vi "main.vi"() -> ()   [LabVIEW 2010]
uses:
  <vilib>/Platform/TimedLoop/XDataNode/XDataNode.xnode
  <vilib>/Platform/TimedLoop/XDataNode/nitl_modes.ctl
  <vilib>/Platform/TimedLoop/XDataNode/XDNodeRunTimeDep.lvlib
  <vilib>/Platform/TimedLoop/XDataNode/wakeup.ctl
  <vilib>/Platform/TimedLoop/XDataNode/timing_clust.ctl
  <vilib>/eio/EIONode/EIONode.xnode
  common_typedefs/DAC_channel_enable_cluster.ctl
  common_typedefs/DAC_voltage_cluster.ctl
  common_typedefs/DAC_values_cluster.ctl
panel:
  in  "converter box version":i16=2 min=1 max=2
  out "current DAQ values":T1={"DAC channel enable"={"ch0"=TRUE, "ch1"=TRUE, "ch2"=TRUE, "ch3"=TRUE, "ch4"=TRUE, "ch5"=TRUE, "ch6"=TRUE}, "DAC voltage"={"ch0"=0, "ch1"=0, "ch2"=0, "ch3"=0, "ch4"=0, "ch5"=0, "ch6"=0}, "offset"=0, "channel index"=0, "bit index"=0, "synch?"=FALSE, "DAC clock"=FALSE, "finished?"=FALSE} {"bit index" min=-1 max=17 step=1; "channel index" max=7 step=1; "offset" max=4095; "DAC voltage"."ch6" max=4095 step=1; "DAC voltage"."ch5" max=4095 step=1; "DAC voltage"."ch4" max=4095 step=1; "DAC voltage"."ch3" max=4095 step=1; "DAC voltage"."ch2" max=4095 step=1; "DAC voltage"."ch1" max=4095 step=1; "DAC voltage"."ch0" max=4095 step=1}
  in  "DAC values in":T1={"DAC channel enable"={"ch0"=TRUE, "ch1"=TRUE, "ch2"=TRUE, "ch3"=TRUE, "ch4"=TRUE, "ch5"=TRUE, "ch6"=TRUE}, "DAC voltage"={"ch0"=0, "ch1"=0, "ch2"=0, "ch3"=0, "ch4"=0, "ch5"=0, "ch6"=0}, "offset"=0, "channel index"=0, "bit index"=0, "synch?"=FALSE, "DAC clock"=FALSE, "finished?"=FALSE} {"bit index" min=-1 max=17 step=1; "channel index" max=7 step=1; "offset" max=4095; "DAC voltage"."ch6" max=4095 step=1; "DAC voltage"."ch5" max=4095 step=1; "DAC voltage"."ch4" max=4095 step=1; "DAC voltage"."ch3" max=4095 step=1; "DAC voltage"."ch2" max=4095 step=1; "DAC voltage"."ch1" max=4095 step=1; "DAC voltage"."ch0" max=4095 step=1}
  in  "dataAndControlResetButton":bool
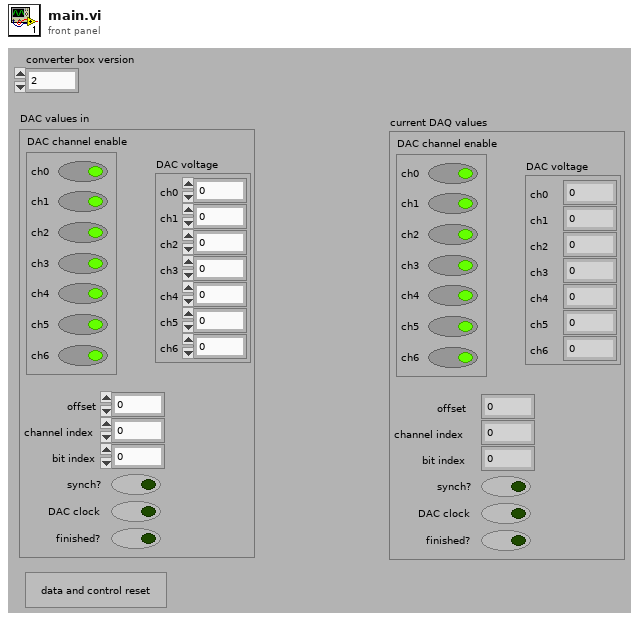
[diagram p1: front panel]
types:
  T1 = typedef "DAC_values_cluster.ctl" = cluster{"DAC channel enable":T2, "DAC voltage":T3, "offset":u16, "channel index":u16, "bit index":i32, "synch?":bool, "DAC clock":bool, "finished?":bool}
  T2 = typedef "DAC_channel_enable_cluster.ctl" = cluster{"ch0":bool, "ch1":bool, "ch2":bool, "ch3":bool, "ch4":bool, "ch5":bool, "ch6":bool}
  T3 = typedef "DAC_voltage_cluster.ctl" = cluster{"ch0":u16, "ch1":u16, "ch2":u16, "ch3":u16, "ch4":u16, "ch5":u16, "ch6":u16}
  T4 = typedef "XDNodeRunTimeDep.lvlib/timing_clust.ctl" = cluster{"Expected End [f-1]":u64, "Actual End [f-1]":u64, "Finished Late? [f-1]":bool, "Expected End [i-1]":u64, "Actual End [i-1]":u64, "Finished Late? [i-1]":bool, "Expected Start [i]":u64, "Actual Start [i]":u64, "Expected Start [f]":u64, "Actual Start [f]":u64, "Source Name":string, "Structure Name":string, "Period":i64, "Deadline":i64, "Offset":i64, "Start":i64, "Priority":i32, "Timeout":i32, "Mode":T5, "Wakeup Reason":T6, "Error":errorcluster, "Source Type":string, "Secondary Source Type":string, "Global End Time":u64, "Global Start Time":u64, "Frame Duration":u64, "Iteration Duration":u64, "Assigned CPU":i32, "I/O Scan Engine Mode":u32}
  T5 = typedef "XDNodeRunTimeDep.lvlib/nitl_modes.ctl" = enum32{"No Change", "Process missed periods, maintain original phase", "Discard missed periods, maintain original phase", "Process missed periods, ignore original phase", "Discard missed periods, ignore original phase"}
  T6 = typedef "XDNodeRunTimeDep.lvlib/wakeup.ctl" = enum32{"Normal", "Aborted", "Asynchronous wakeup", "Timing source error", "Timed loop error", "Timeout"}
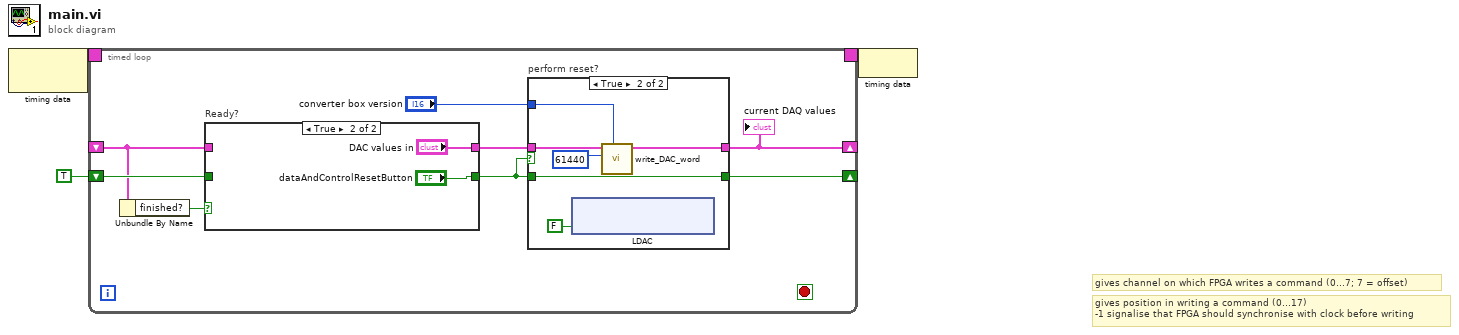
[diagram p0: block diagram]
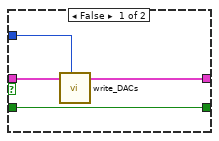
[diagram p2: hidden frame]
diagram:
  # "gives channel on which FPGA writes a command (0...7; 7 = offset)"
  # "gives position in writing a command (0...17)\n-1 signalise that FPGA should synchronise with clock before writing"
  n1 = node-c288() -> (w3:T4)  [unwired: 1 in]
  n2 = timed-loop {
    timing: w3 -> [_]
    timing-out: [_] -> w2
    shift-right: [w10] -> _
    shift-left: TRUE -> [w11]
    shift-right: [w4] -> _
    shift-left: _ -> [w7]
    stop <- _ stop-if-true
    n3 = Unbundle By Name(w7) -> ("finished?"=w6:bool)
    n4 = case "Ready?" shown="True" w6 {
      tunnel: w11 -> [w23 _]
      tunnel: [w23 "dataAndControlResetButton"] -> w9
      tunnel: [w22 "DAC values in"] -> w8
      tunnel: w7 -> [w22 _]
      frame False {
      }
      frame True {
      }
    }
    n5 = case "perform reset?" shown="True" w9 {
      tunnel: [w15 w21] -> w10
      tunnel: w9 -> [w15 w21]
      tunnel: w8 -> [w14 w18]
      tunnel: [w13 w17] -> w4
      tunnel: "converter box version" -> [w12 w16]
      frame False {
        n6 = call "write_DACs.vi"("converter box version"=w12, "DAC values in"=w14) -> ("DAQ values out"=w13:T1)  [unwired: 9 in]
      }
      frame True {
        n7 = xnode "LDAC"("Connector1/DIO32"=FALSE ("LDAC")) -> ()  [unwired: 1 in, 1 out]
        n8 = call "write_DAC_word.vi"("converter box version"=w16, "U16 data number"=u16 61440 ("number"), "DAC values in"=w18) -> ("DAC values out"=w17:T1)  [unwired: 8 in]
      }
    }
    "current DAQ values" <- w4
  }
  n9 = node-c288(w2) -> ()
